vi "TGA read.vi"(11 "file path (dialog if empty)":path=path "C:/Users/Administrator/Desktop/4f1f1f767bbf47ebb845cae200a72e59LX180906650TGA.txt") -> (2 "rawData":string[][](array[string]), 3 "dataCheckOK":bool)   [LabVIEW 2011]
uses:
  <vilib>/Utility/file.llb/Read From Spreadsheet File (string).vi
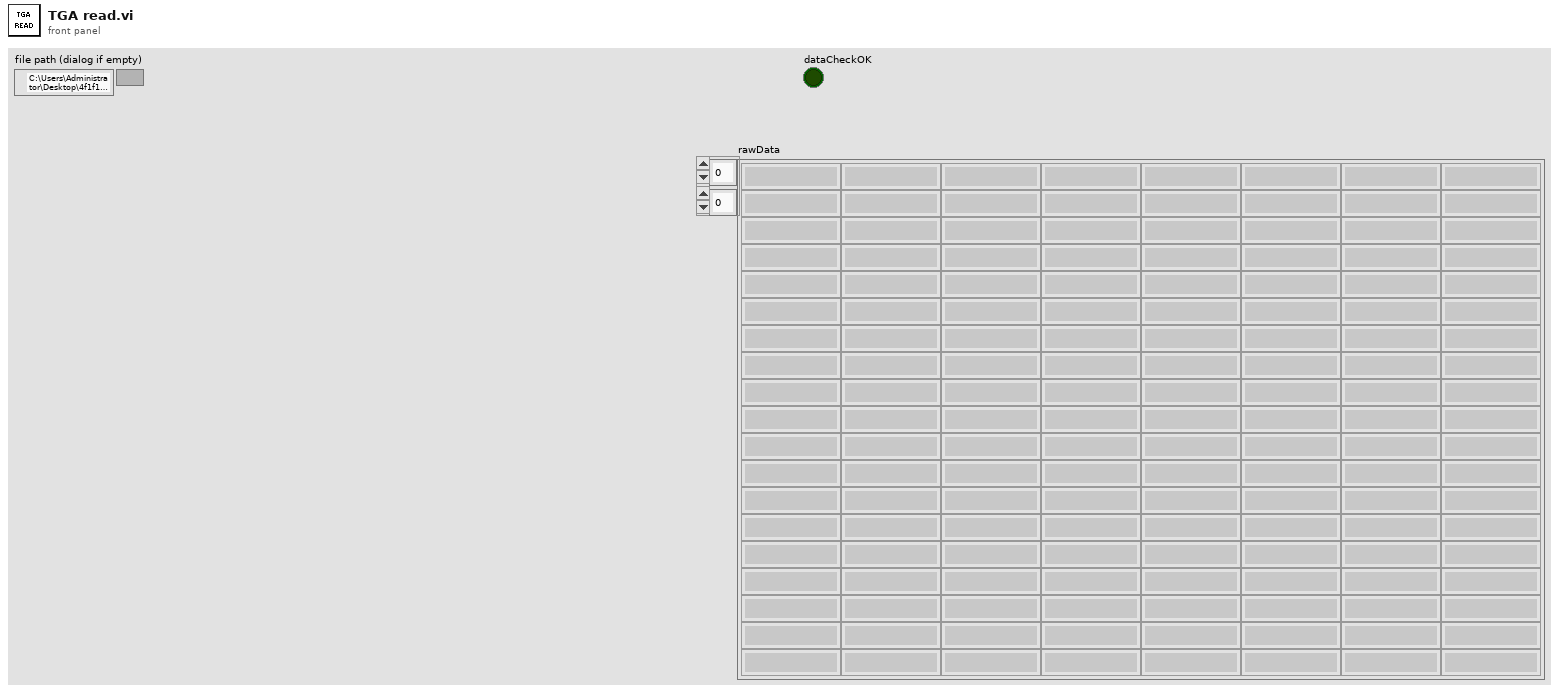
[diagram p1: front panel]
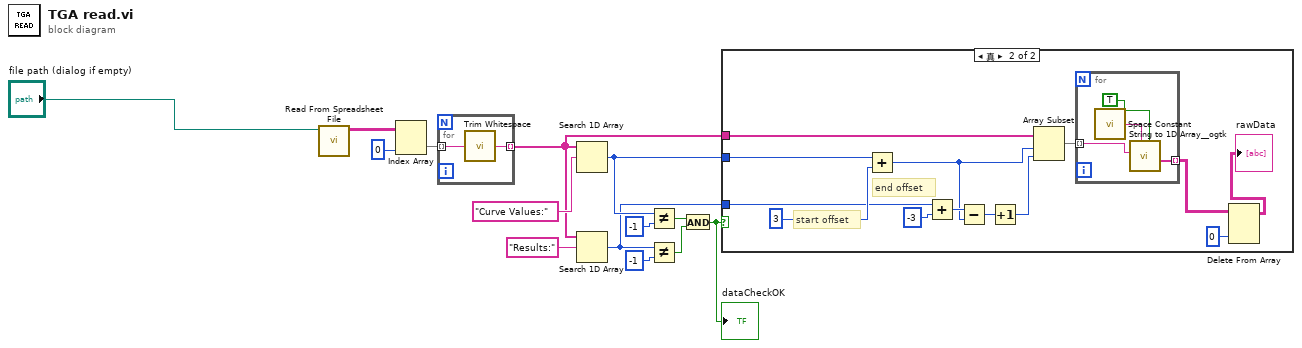
[diagram p0: block diagram]
diagram:
  n1 = call-poly <vilib>:"Read From Spreadsheet File.vi"("file path (dialog if empty)"="file path (dialog if empty)") -> ("all rows"=w14:string[][])  [unwired: 6 in, 4 out]
  n2 = Index Array(array=w14, index (col)=0 ("索引 (行)")) -> (element=w12:string[])  [unwired: 1 in]
  n3 = for {
    tunnel: w12 -> [w16] mode=indexing
    tunnel: [w15] -> w1 mode=indexing
    n4 = call <vilib>:"Trim Whitespace.vi"("string"=w16) -> ("trimmed string"=w15:string)  [unwired: 1 in]
  }
  n5 = Search 1D Array(1D array=w1, element="Curve Values:" ("元素")) -> (index of element=w3:i32)  [unwired: 1 in]
  n6 = Search 1D Array(1D array=w1, element="Results:" ("元素")) -> (index of element=w2:i32)  [unwired: 1 in]
  n7 = Not Equal?(x=w3, y=-1) -> (x != y?=w6:bool)
  n8 = Not Equal?(x=w2, y=-1) -> (x != y?=w5:bool)
  n9 = And(x=w6, y=w5) -> (x .and. y?=w4:bool)
  "dataCheckOK" <- w4
  n10 = case shown="真" w4 {
    tunnel: w3 -> [_ w29]
    tunnel: w2 -> [_ w27]
    tunnel: w1 -> [_ w25]
    frame False {
    }
    frame True {
      # "end offset"
      # "start offset"
      n11 = Add(x=w29, y=3) -> (x+y=w23:i32)
      n12 = Add(x=w27, y=-3) -> (x+y=w24:i32)
      n13 = Subtract(x=w24, y=w23) -> (x-y=w22:i32)
      n14 = Increment(x=w22) -> (x+1=w21:i32)
      n15 = Array Subset(array=w25, index=w23, length=w21) -> (w20:string[])
      n16 = for {
        tunnel: w20 -> [w33] mode=indexing
        tunnel: [w32] -> w19 mode=indexing
        n17 = call <vilib>:"Space Constant.vi"() -> ("String"=w30:string)
        n18 = call <userlib>:"String to 1D Array__ogtk.vi"("ignore duplicate delimiters? (F=No)"=TRUE, "delimiter (Tab)"=w30, "string"=w33) -> ("Array of Strings"=w32:string[])  [unwired: 8 in]
      }
      n19 = Delete From Array(array=w19, index (col)=0 ("禁用的索引 (列)")) -> (array with subset deleted=→"rawData":string[][])  [unwired: 2 in, 1 out]
    }
  }
